vi "Rejection_SQL_data_fetch.vi"(6 "error constant":errorcluster, 7 "Cycle Data":T1={"CID"="", "Comm Stat"=FALSE, "Input"=[FALSE, FALSE, FALSE, FALSE, FALSE], "ip address's"="", "CYCLE COUNT"=0, "REJECTION COUNT"=0, "PRODUCT_CODE"=0, "ALARAM"=[FALSE, FALSE, FALSE, FALSE, FALSE, FALSE, FALSE, FALSE], "OUTPUT"=[FALSE, FALSE, FALSE, FALSE, FALSE], "PARTS PER HOUR"=0, "MR Retn Tmr"=0.0, "Holding Tmr"=0.0, "1st Pressure"=0.0, "2nd Pressure"=0.0}, 8 "Current Shift":i32, 9 "connection reference":T2) -> (0 "error out 3":errorcluster, 2 "Refnum out 2":T2, 3 "MAX Rejection ID":i32)   [LabVIEW 2017]
uses:
  <vilib>/addons/database/Connection.llb/Conn ObjectReference.ctl
  Control/Main_Data.ctl
  <vilib>/addons/database/Connection.llb/Conn Execute.vi
  <vilib>/addons/database/Recordset.llb/Rec Fetch Recordset Data (R).vi
  <vilib>/addons/database/Recordset.llb/Rec Destroy - Connection.vi
  <vilib>/addons/database/NI_Database_API.lvlib
panel:
  out "SHIFT":i32
  out "DATE":string
  out "recordset data":variant[][](array[variant])
  out "resulting string":string
  out "REJ COUNT":i32
  out "REJECTION COUNT":i32
  out "TABLE NAME":string
  out "error out":errorcluster
  # "Rejection check and add to DataBase"
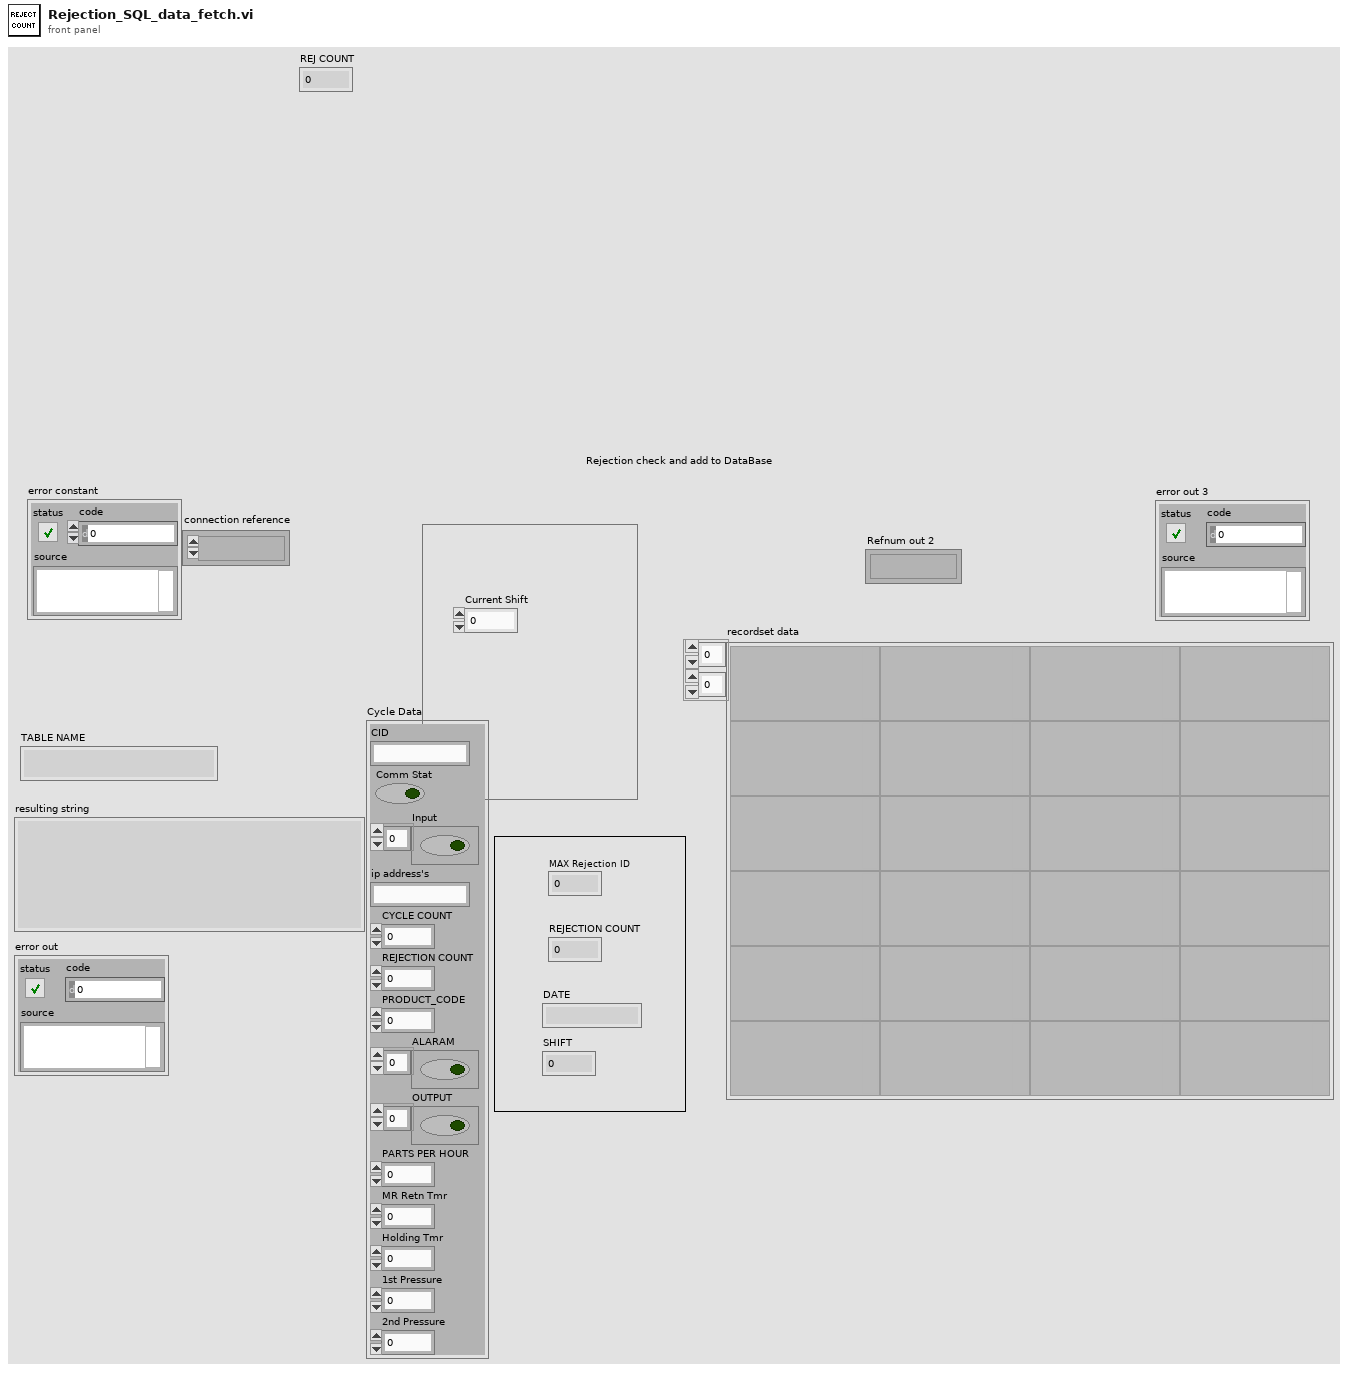
[diagram p1: front panel]
types:
  T1 = typedef "Main_Data.ctl" = cluster{"CID":string, "Comm Stat":bool, "Input":bool[], "ip address's":string, "CYCLE COUNT":u32, "REJECTION COUNT":u32, "PRODUCT_CODE":i16, "ALARAM":bool[], "OUTPUT":bool[], "PARTS PER HOUR":i16, "MR Retn Tmr":dbl, "Holding Tmr":dbl, "1st Pressure":dbl, "2nd Pressure":dbl}
  T2 = typedef "NI_Database_API.lvlib/Conn ObjectReference.ctl" = refnum<k1>
  T3 = typedef "NI_Database_API.lvlib/Rec ObjectReference.ctl" = refnum<k1>
  T4 = typedef "LVDateTimeRec.ctl" = cluster{"fractional second":dbl, "second":i32, "minute":i32, "hour":i32, "day of month":i32, "month":i32, "year":i32, "day of week":i32, "day of year":i32, "DST":i32}
  T5 = cluster{i32, "CID":string, "REJECTION COUNT":u32, "Current Shift":i32, "date/time string":string, "Date String":string, string, string}
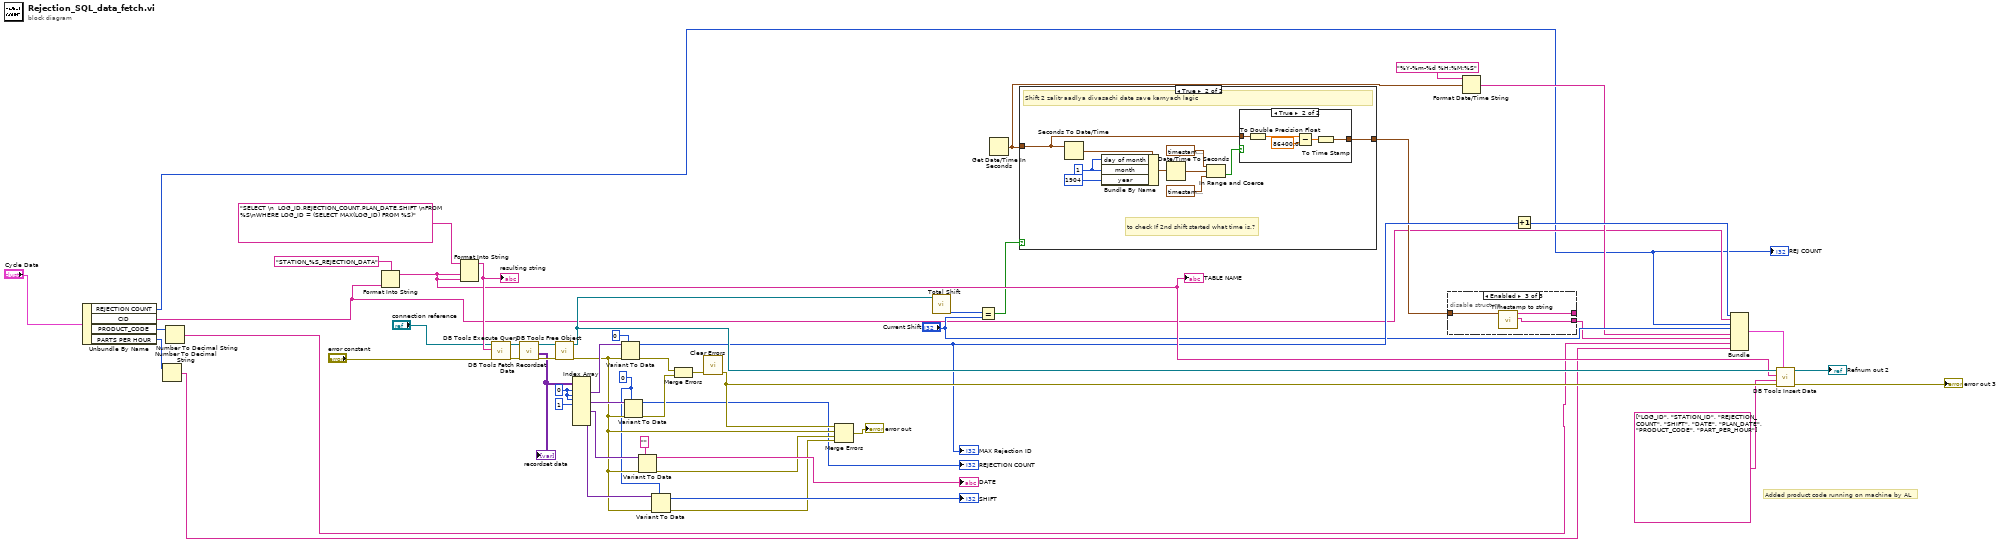
[diagram p0: block diagram]
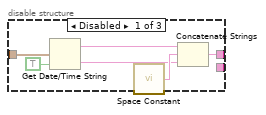
[diagram p2: hidden frame]
diagram:
  w26 = 0
  w42 = 0 ("index (row)")
  # "Added product code running on machine by AL"
  n1 = Unbundle By Name("Cycle Data") -> ("REJECTION COUNT"=w3:u32, "CID"=w4:string, "PRODUCT_CODE"=w7:i16, "PARTS PER HOUR"=w6:i16)
  "REJ COUNT" <- w3
  n2 = Number To Decimal String(number=w6) -> (decimal integer string=w1:string)  [unwired: 1 in]
  n3 = Number To Decimal String(number=w7) -> (decimal integer string=w2:string)  [unwired: 1 in]
  n4 = Format Into String(format string="STATION_%S_REJECTION_DATA" ("SQL query"), w4) -> (resulting string=w34:string)  [unwired: 2 in, 1 out]
  "TABLE NAME" <- w34
  n5 = Format Into String(format string="SELECT \n  LOG_ID,REJECTION_COUNT,PLAN_DATE,SHIFT \nFROM %S\nWHERE LOG_ID = (SELECT MAX(LOG_ID) FROM %S)" ("SQL query"), w34, w34) -> (resulting string=w46:string)  [unwired: 2 in, 1 out]
  "resulting string" <- w46
  n6 = call-poly <vilib>:"DB Tools Execute Query.vi"("error in (no error)"="error constant", "SQL query"=w46, "connection reference"="connection reference") -> ("error out"=w50:errorcluster, "recordset reference"=w51:T3)  [unwired: 5 in]
  n7 = call-poly <vilib>:"DB Tools Fetch Recordset Data.vi"("error in (no error)"=w50, "recordset reference"=w51) -> ("error out"=w49:errorcluster, "recordset data"=w32:variant[][], "recordset reference out"=w52:T3)  [unwired: 3 in]
  "recordset data" <- w32
  n8 = call-poly <vilib>:"DB Tools Free Object.vi"("error in (no error)"=w49, "recordset reference"=w52) -> ("error out"=w27:errorcluster, "connection reference"=w35:T2)  [unwired: 8 in]
  n9 = Index Array(array=w32, index (row) #1=w42, index (col) #1=w42, index (row) #2=w42, index (col) #2=1 ("index (row)")) -> (element #1=w47:variant, element #2=w41:variant, element #3=w31:variant, element #4=w28:variant)  [unwired: 4 in]
  n10 = Variant To Data(error in=w27, type=0, Variant=w47) -> (data=w33:i32, error out=w53:errorcluster)
  "MAX Rejection ID" <- w33
  n11 = Variant To Data(error in=w27, type=w26, Variant=w41) -> (data=→"REJECTION COUNT":i32, error out=w39:errorcluster)
  n12 = Variant To Data(error in=w27, type="", Variant=w31) -> (data=→"DATE":string, error out=w24:errorcluster)
  n13 = Variant To Data(error in=w27, type=w26, Variant=w28) -> (data=→"SHIFT":i32, error out=w23:errorcluster)
  n14 = Merge Errors(w53, w39) -> (w40:errorcluster)
  n15 = call <vilib>:"Clear Errors.vi"("error in (no error)"=w40) -> ("error out"=w36:errorcluster)  [unwired: 5 in, 1 out]
  n16 = Merge Errors(w36, w27, w24, w23) -> (→"error out":errorcluster)
  n17 = call "Total Shift.vi"("connection reference"=w35) -> ("Total Shifts"=w19:i32)  [unwired: 9 in, 1 out]
  n18 = Equal?(x=w19, y="Current Shift") -> (x = y?=w20:bool)
  n19 = Get Date/Time In Seconds() -> (seconds since 1Jan1904=w9:timestamp)
  n20 = case shown="True" w20 {
    tunnel: w9 -> [w54 w55]
    tunnel: [w54 w56] -> w10
    frame False {
    }
    frame True {
      w61 = 1 ("day of month")
      # "to check If 2nd shift started what time is.?"
      # "Shift 2 zalitr aadlya divasachi date save karnyach lagic"
      n21 = Seconds To Date/Time(time stamp (now)=w55) -> (date time rec=w62:T4)  [unwired: 1 in]
      n22 = Bundle By Name(cluster=w62, "day of month"=w61, "month"=w61, "year"=1904) -> (w64:T4)
      n23 = Date/Time To Seconds(2:w64) -> (0:w60:timestamp)  [unwired: 1 in]
      n24 = In Range and Coerce(upper limit=timestamp(5399 s since 1904-01-01), x=w60, lower limit=timestamp(-19800 s since 1904-01-01)) -> (In Range?=w57:bool)  [unwired: 1 out]
      n25 = case shown="True" w57 {
        tunnel: [w65 w67] -> w56
        tunnel: w55 -> [w65 w66]
        frame False {
        }
        frame True {
          n26 = To Double Precision Float(number=w66) -> (double precision float=w70:dbl)
          n27 = Subtract(x=w70, y=86400.0) -> (x-y=w68:dbl)
          n28 = To Time Stamp(1:w68) -> (0:w67:timestamp)
        }
      }
    }
  }
  n29 = disable-structure shown="Enabled" {
    disable-tunnel: w10 -> [w76 w77 w80]
    disable-tunnel: [w72 w77 w79] -> _
    disable-tunnel: [_ _ w78] -> w17
    frame Disabled {
      n30 = Get Date/Time String(seconds (now)=w76, want seconds? (F)=TRUE) -> (date string=w73:string, time string=w74:string)  [unwired: 1 in]
      n31 = call <vilib>:"Space Constant.vi"() -> ("String"=w75:string)
      n32 = Concatenate Strings(w73, w75, w74) -> (w72:string)
    }
    frame Disabled {
    }
    frame Enabled {
      n33 = call "Timestamp to string.vi"("time stamp"=w80) -> ("Date String"=w78:string, "date/time string"=w79:string)  [unwired: 8 in, 1 out]
    }
  }
  n34 = Format Date/Time String(time format string (%c)="%Y-%m-%d %H:%M:%S", seconds (now)=w9) -> (date/time string=w8:string)  [unwired: 1 in]
  n35 = Increment(x=w33) -> (x+1=w21:i32)
  n36 = Bundle(w21, "CID"=w4, "REJECTION COUNT"=w3, "Current Shift"="Current Shift", "date/time string"=w8, "Date String"=w17, w2, w1) -> (w22:T5)  [unwired: 1 in]
  n37 = call <vilib>:"DB Tools Insert Data.vi"("data"=w22, "error in (no error)"=w36, "columns"=string[] ["LOG_ID", "STATION_ID", "REJECTION_COUNT", "SHIFT", "DATE", "PLAN_DATE", "PRODUCT_CODE", "PART_PER_HOUR"], "table"=w34, "connection reference"=w35) -> ("error out"=→"error out 3":errorcluster, "connection reference out"=→"Refnum out 2":T2)  [unwired: 5 in]
